vi "Renishaw-XL80_SetResetCompensationMethod.vi"(8 "error in (no error)":errorcluster, 11 "Renishaw-XL80 in":refnum<class "Renishaw-XL80.lvclass">) -> (0 "error out":errorcluster, 3 "Renishaw-XL80 out":refnum<class "Renishaw-XL80.lvclass">)   [LabVIEW 2024, in "Renishaw-XL80.lvclass"]
doc: "This method switches auto-compensation off, returns lambda to its NTP value, and the material compensation factor to 1.\n\nDefinition\nHRESULTResetCompensation();\nParameters\nNone\n\nComments\nThis method always succeeds and returns an HRESULT of S_OK.\n\nIf the client wishes to be compatible with the behaviour of Laser10, then whenever the MeasurementMode is changed to MEASUREMENT_ANGULAR, MEASUREMENT_STRAIGHTNESS_SHORT, or MEASUREMENT_STRAIGHTNESS_LONG then this method should be called in order to turn compensation off."
uses:
  Renishaw-XL80.lvclass
  Renishaw-XL80.lvclass/Renishaw-XL80.ctl
  D:/A.C.M/Example CSharp_64/bin/Debug/Interop.DX10SDKADAPTORLib.dll
  Example CSharp_64/bin/Debug/Interop.DX10SDKADAPTORLib.dll
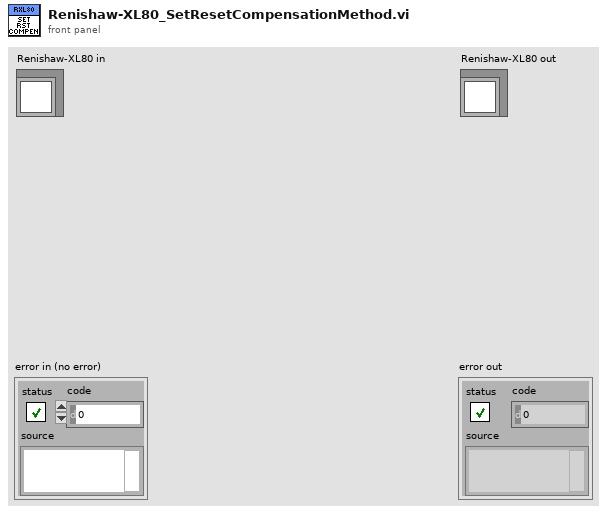
[diagram p1: front panel]
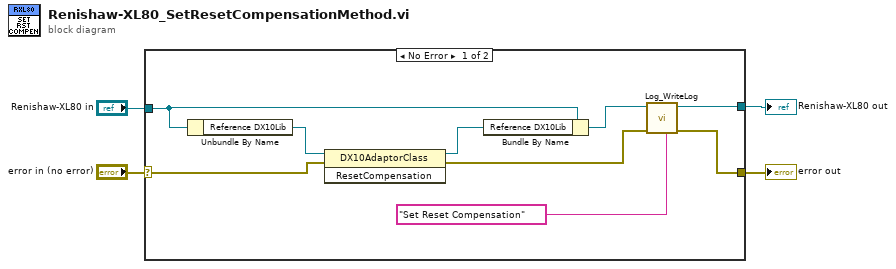
[diagram p0: block diagram]
diagram:
  n1 = case shown="No Error" "error in (no error)" {
    selector: "error in (no error)" -> [w10 w15]
    tunnel: [w6 w15] -> w3
    tunnel: [w9 w14] -> w1
    tunnel: "Renishaw-XL80 in" -> [w12 w14]
    frame No Error {
      n2 = Unbundle By Name(w12) -> ("Reference DX10Lib"=w13:refnum<k24>)
      n3 = invoke class="DX10AdaptorClass" method="ResetCompensation"(reference=w13, error in=w10) -> (reference out=w11:refnum<k24>, error out=w7:errorcluster)  [unwired: 1 in, 1 out]
      n4 = Bundle By Name(cluster=w12, "Reference DX10Lib"=w11) -> (w8:refnum<class "Renishaw-XL80.lvclass">)
      n5 = call-dynamic "Log_WriteLog.vi"("Additional text"="Set Reset Compensation", "error in (no error)"=w7, "Log in"=w8) -> ("error out"=w6:errorcluster, "Log out"=w9:refnum<class "Renishaw-XL80.lvclass">)  [unwired: 7 in]
    }
    frame Error {
    }
  }
  "error out" <- w3
  "Renishaw-XL80 out" <- w1
